vi "Write PAS DVR.vi"(8 "error in (no error)":errorcluster, 10 "PAS DVR":refnum<data-value>, 11 "Collect Data in":refnum<class "Collect Data.lvclass">) -> (0 "error out":errorcluster, 3 "Collect Data out":refnum<class "Collect Data.lvclass">)   [LabVIEW 2015, in "Collect Data.lvclass"]
uses:
  Collect Data.lvclass
  Data/cPAS Data.lvclass
  Collect Data.lvclass/Collect Data.ctl
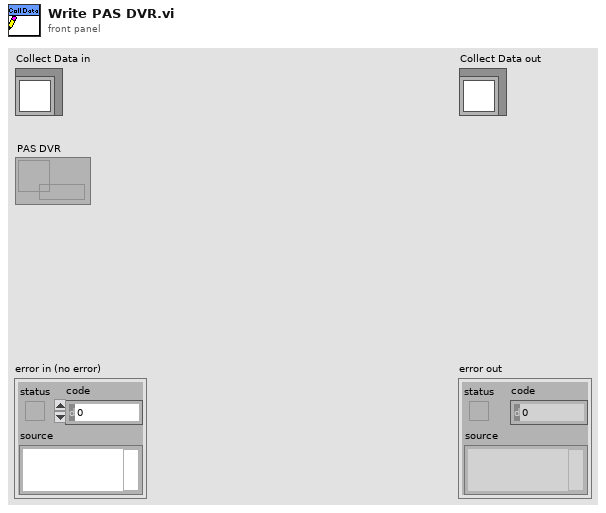
[diagram p1: front panel]
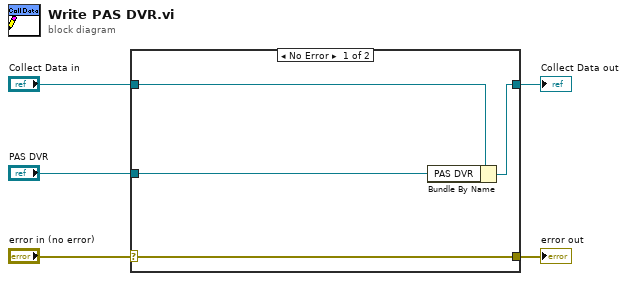
[diagram p0: block diagram]
diagram:
  n1 = case shown="No Error" "error in (no error)" {
    selector: "error in (no error)" -> [w9 w10]
    tunnel: [w9 w10] -> w4
    tunnel: [w7 w11] -> w2
    tunnel: "Collect Data in" -> [w8 w11]
    tunnel: "PAS DVR" -> [w6 _]
    frame No Error {
      n2 = Bundle By Name(cluster=w8, "PAS DVR"=w6) -> (w7:refnum<class "Collect Data.lvclass">)
    }
    frame Error {
    }
  }
  "error out" <- w4
  "Collect Data out" <- w2
